vi "Timestamp to ISO8601 Year.vi"(9 "UTC? (F)":bool, 11 "Timestamp (now)":timestamp) -> (1 "is Leap Year?":bool, 3 "year":i32)   [LabVIEW 2018]
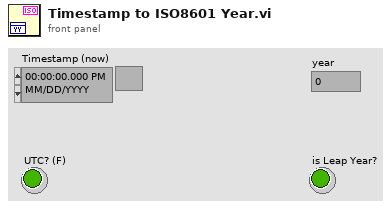
[diagram p1: front panel]
types:
  T1 = typedef "LVDateTimeRec.ctl" = cluster{"fractional second":dbl, "second":i32, "minute":i32, "hour":i32, "day of month":i32, "month":i32, "year":i32, "day of week":i32, "day of year":i32, "DST":i32}
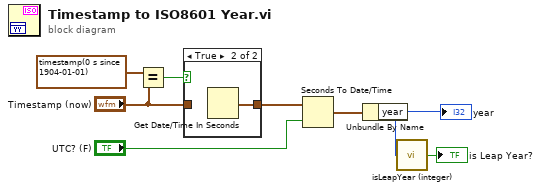
[diagram p0: block diagram]
diagram:
  n1 = Equal?(x=timestamp(0 s since 1904-01-01), y="Timestamp (now)") -> (x = y?=w5:bool)
  n2 = case shown="True" w5 {
    tunnel: [w9 w10] -> w3
    tunnel: "Timestamp (now)" -> [w9 _]
    frame False {
    }
    frame True {
      n3 = Get Date/Time In Seconds() -> (seconds since 1Jan1904=w10:timestamp)
    }
  }
  n4 = Seconds To Date/Time(time stamp (now)=w3, to UTC (F)="UTC? (F)") -> (date time rec=w7:T1)
  n5 = Unbundle By Name(w7) -> ("year"=w2:i32)
  "year" <- w2
  n6 = call "isLeapYear (integer).vi"("Year (0: this year)"=w2) -> ("is Leap Year?"=→"is Leap Year?":bool)  [unwired: 8 in]
